vi "Analysis.Result Summaries, Generate Pareto_V2a.vi"(9 "Type":enum16{"All", "FP", "LP"}(ring), 11 "ResultSum":T1[](array[typedef])) -> (3 "FP Pareto":string[][](table))   [LabVIEW 2024]
uses:
  Analysis.Fail Paredo Gen Input_V2.ctl
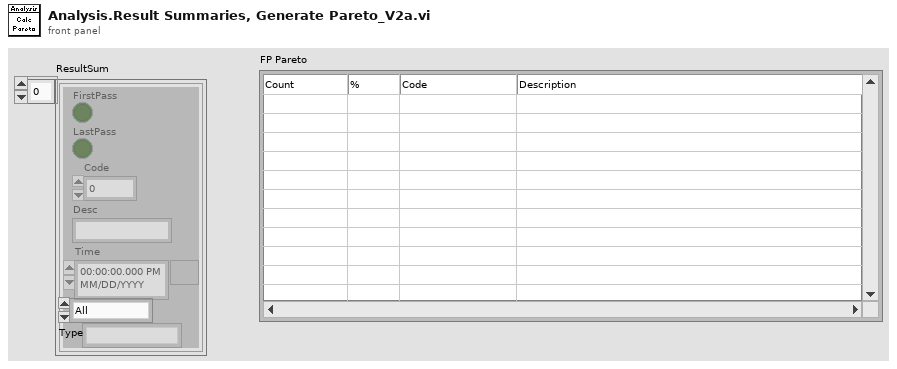
[diagram p1: front panel]
types:
  T1 = typedef "Analysis.Fail Paredo Gen Input_V2.ctl" = cluster{"FirstPass":bool, "LastPass":bool, "Code":i32, "Desc":string, "Time":timestamp, "Loc":string}
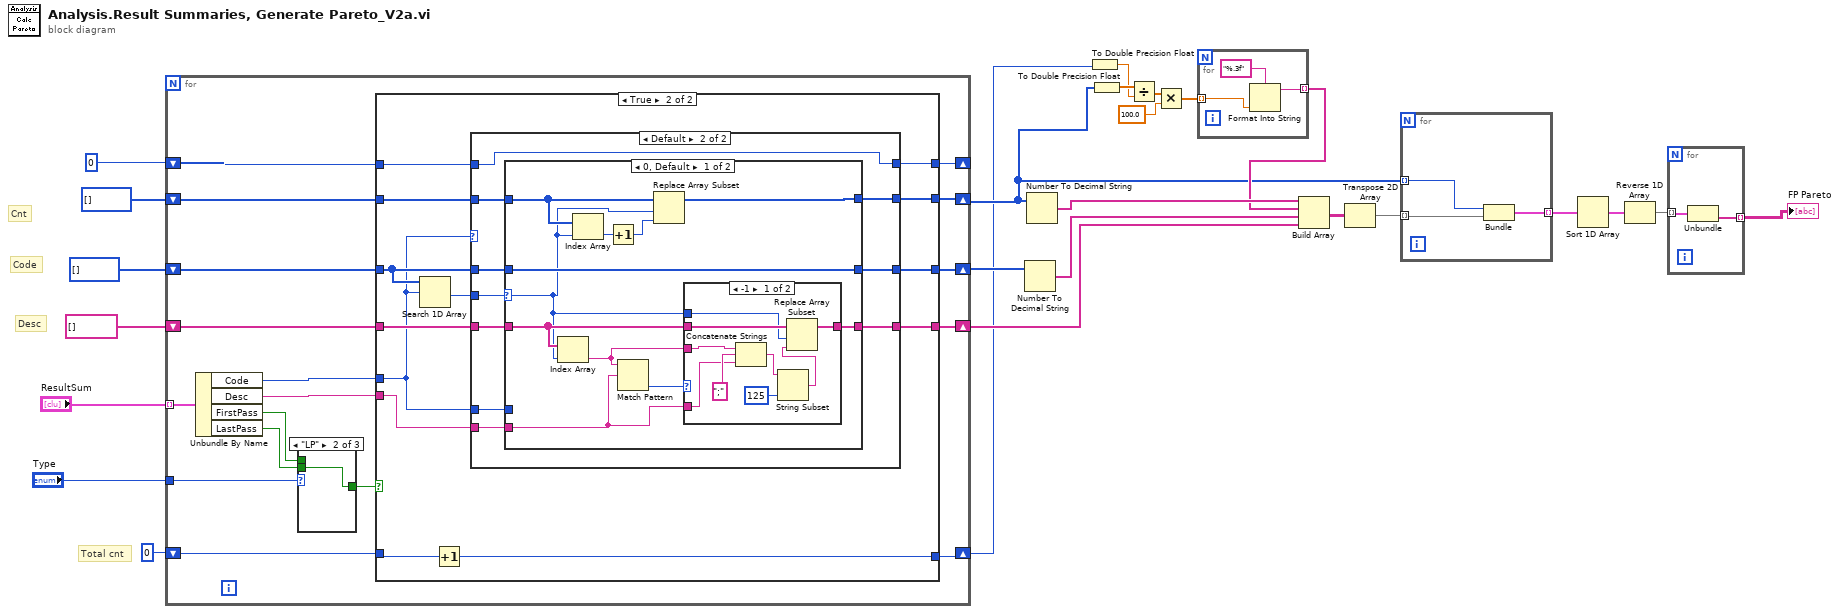
[diagram p0: block diagram]
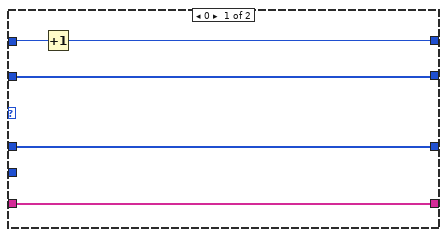
[diagram p3: hidden frame]
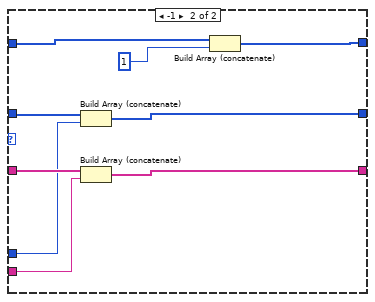
[diagram p5: hidden frame]
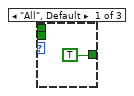
[diagram p6: hidden frame]
diagram:
  # "Total cnt"
  # "Desc"
  # "Code"
  # "Cnt"
  n1 = for {
    shift-right: [w39] -> w9
    shift-left: i32[] [] -> [w42]
    shift-right: [w38] -> w6
    shift-left: i32[] [] -> [w41]
    shift-right: [w37] -> w22
    shift-left: string[] [] -> [w40]
    tunnel: "ResultSum" -> [w34] mode=indexing
    shift-right: [w35] -> _
    shift-left: 0 ("Numeric") -> [w36]
    shift-right: [w26] -> w1
    shift-left: 0 ("Numeric") -> [w27]
    tunnel: "Type" -> [w31]
    n2 = Unbundle By Name(w34) -> ("Code"=w33:i32, "Desc"=w32:string, "FirstPass"=w30:bool, "LastPass"=w29:bool)
    n3 = case shown="\"LP\"" w31 {
      tunnel: w30 -> [_ _ w108]
      tunnel: w29 -> [_ w107 _]
      tunnel: [TRUE w107 w108] -> w28
      frame "All", Default {
      }
      frame "LP" {
      }
      frame "FP" {
      }
    }
    n4 = case shown="True" w28 {
      tunnel: w42 -> [w45 w59]
      tunnel: w41 -> [w44 w58]
      tunnel: w40 -> [w43 w57]
      tunnel: [w45 w56] -> w39
      tunnel: [w44 w55] -> w38
      tunnel: [w43 w54] -> w37
      tunnel: w36 -> [w46 w53]
      tunnel: [w46 w52] -> w35
      tunnel: w33 -> [_ w51]
      tunnel: w32 -> [_ w50]
      tunnel: w27 -> [w47 w49]
      tunnel: [w47 w48] -> w26
      frame False {
      }
      frame True {
        n5 = Search 1D Array(1D array=w58, element=w51) -> (index of element=w60:i32)  [unwired: 1 in]
        n6 = Increment(x=w49) -> (x+1=w48:i32)
        n7 = case shown="Default" w51 {
          tunnel: w60 -> [_ w75]
          tunnel: w59 -> [w65 w74]
          tunnel: w58 -> [w64 w73]
          tunnel: w57 -> [w63 w72]
          tunnel: [w65 w71] -> w56
          tunnel: [w64 w70] -> w55
          tunnel: [w63 w69] -> w54
          tunnel: w51 -> [_ w68]
          tunnel: w50 -> [_ w67]
          tunnel: w53 -> [w62 w66]
          tunnel: [w61 w66] -> w52
          frame 0 {
            n8 = Increment(x=w62) -> (x+1=w61:i32)
          }
          frame Default {
            n9 = case shown="0, Default" w75 {
              selector: w75 -> [w76 _]
              tunnel: w74 -> [w85 w102]
              tunnel: w73 -> [w82 w104]
              tunnel: w72 -> [w80 w105]
              tunnel: [w86 w101] -> w71
              tunnel: [w82 w100] -> w70
              tunnel: [w79 w99] -> w69
              tunnel: w68 -> [_ w97]
              tunnel: w67 -> [w77 w98]
              frame 0, Default {
                n10 = Index Array(array=w80, index=w76) -> (element=w78:string)
                n11 = Index Array(array=w85, index=w76) -> (element=w84:i32)
                n12 = Increment(x=w84) -> (x+1=w83:i32)
                n13 = Match Pattern(string=w78, regular expression=w77) -> (offset past match=w81:i32)  [unwired: 1 in, 3 out]
                n14 = Replace Array Subset(array=w85, new element=w83, index=w76) -> (w86:i32[])
                n15 = case shown="-1" w81 {
                  tunnel: w80 -> [w94 w96]
                  tunnel: [w95 w96] -> w79
                  tunnel: w78 -> [w93 _]
                  tunnel: w77 -> [w91 _]
                  tunnel: w76 -> [w90 _]
                  frame -1 {
                    n16 = Concatenate Strings(w93, ";", w91) -> (w89:string)
                    n17 = String Subset(string=w89, length (rest)=125 ("length (rest)")) -> (substring=w87:string)  [unwired: 1 in]
                    n18 = Replace Array Subset(array=w94, new element=w87, index=w90) -> (w95:string[])
                  }
                  frame Default {
                  }
                }
              }
              frame -1 {
                n19 = Build Array (concatenate)(w104, w97) -> (w100:i32[])
                n20 = Build Array (concatenate)(w105, w98) -> (w99:string[])
                n21 = Build Array (concatenate)(w102, 1) -> (w101:i32[])
              }
            }
          }
        }
      }
    }
  }
  n22 = Number To Decimal String(number=w6) -> (decimal integer string=w5:string[])  [unwired: 1 in]
  n23 = Number To Decimal String(number=w9) -> (decimal integer string=w11:string[])  [unwired: 1 in]
  n24 = To Double Precision Float(number=w1) -> (double precision float=w7:dbl)
  n25 = To Double Precision Float(number=w9) -> (double precision float=w8:dbl[])
  n26 = Divide(x=w8, y=w7) -> (x/y=w12:dbl[])
  n27 = Multiply(x=w12, y=100.0) -> (x*y=w14:dbl[])
  n28 = for {
    tunnel: w14 -> [w110] mode=indexing
    tunnel: [w109] -> w10 mode=indexing
    n29 = Format Into String(format string="%.3f", w110) -> (resulting string=w109:string)  [unwired: 2 in, 1 out]
  }
  n30 = Build Array(w11, w10, w5, w22) -> (w21:string[][])
  n31 = Transpose 2D Array(2D array=w21) -> (transposed array=w20:string[][])
  n32 = for {
    tunnel: w20 -> [w112] mode=indexing
    tunnel: w9 -> [w114] mode=indexing
    tunnel: [w113] -> w18 mode=indexing
    n33 = Bundle("Numeric"=w114, w112) -> (w113:cluster{"Numeric":i32, string[]})  [unwired: 1 in]
  }
  n34 = Sort 1D Array(array=w18) -> (sorted array=w17:cluster{"Numeric":i32, string[]}[])
  n35 = Reverse 1D Array(array=w17) -> (reversed array=w16:cluster{"Numeric":i32, string[]}[])
  n36 = for {
    tunnel: w16 -> [w116] mode=indexing
    tunnel: [w115] -> w15 mode=indexing
    n37 = Unbundle(w116) -> (w115:string[])  [unwired: 1 out]
  }
  "FP Pareto" <- w15
